vi "HEWH_EnviraCom_Main.vi"(1 "Envira is working":refnum<vi>, 4 "Loop Count":refnum<vi>, 6 "State":refnum<vi>, 8 "error in":errorcluster, 9 "Retry Count":refnum<vi>, 11 "Message Queues out":T1) -> (0 "error out":errorcluster)   [LabVIEW 2023]
uses:
  Tenney/support/Message Queue/All Message Queues.ctl
  Tenney/support/Message Queue/Message Cluster.ctl
  FVIR and LDO/support/Message Queue/Enqueue Message (Single).vi
  FVIR and LDO/support/Message Queue/Message Queue.lvlib
  Tenney/support/Message Queue/Tenney Message Queue.lvlib
panel:
  out "Debug":string[](array[string])
  in  "Debug":bool
  out "Loop Count":i32
  # "Debug"
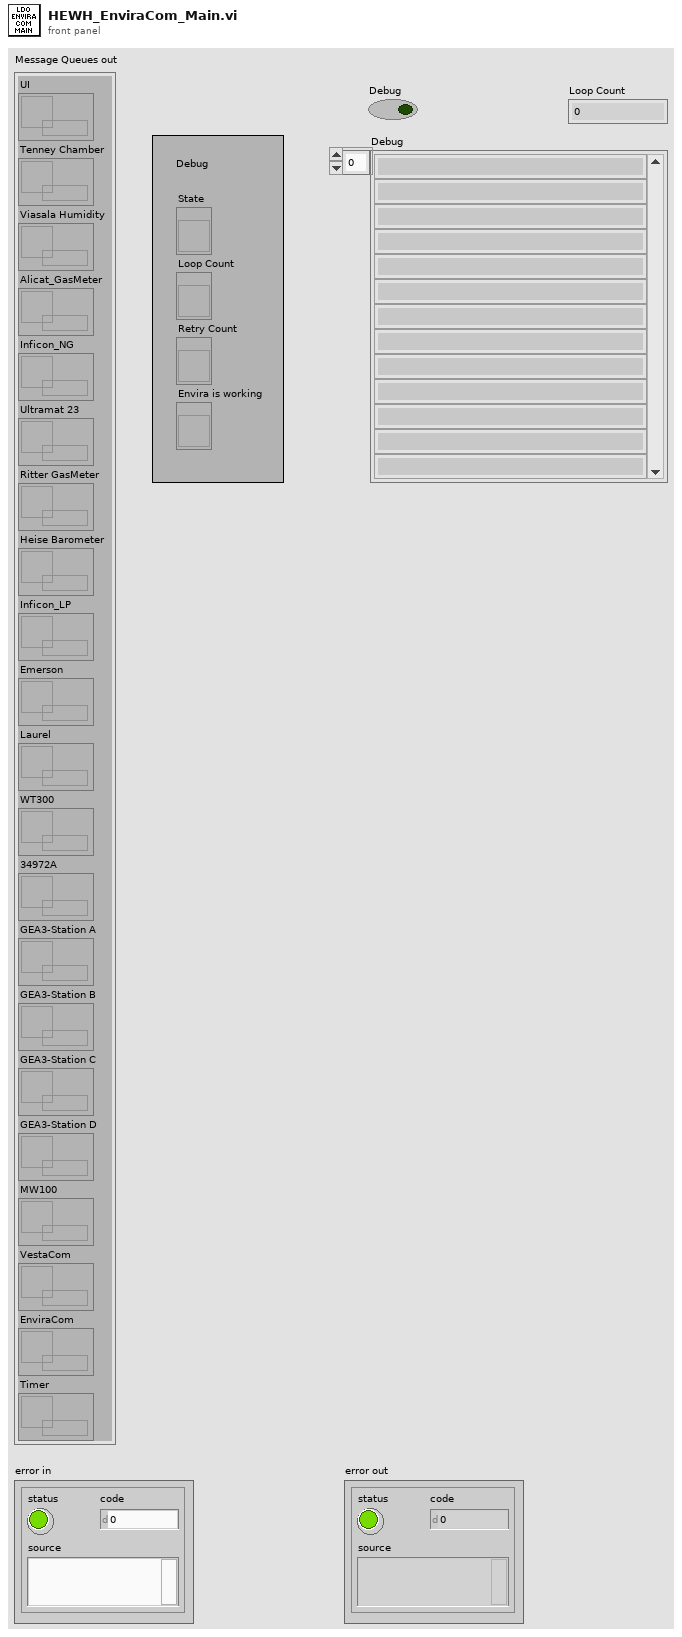
[diagram p1: front panel]
types:
  T1 = typedef "Tenney Message Queue.lvlib/All Message Queues.ctl" = cluster{"UI":refnum<queue>, "Tenney Chamber":refnum<queue>, "Viasala Humidity":refnum<queue>, "Alicat_GasMeter":refnum<queue>, "Inficon_NG":refnum<queue>, "Ultramat 23":refnum<queue>, "Ritter GasMeter":refnum<queue>, "Heise Barometer":refnum<queue>, "Inficon_LP":refnum<queue>, "Emerson":refnum<queue>, "Laurel":refnum<queue>, "WT300":refnum<queue>, "34972A":refnum<queue>, "GEA3-Station A":refnum<queue>, "GEA3-Station B":refnum<queue>, "GEA3-Station C":refnum<queue>, "GEA3-Station D":refnum<queue>, "MW100":refnum<queue>, "VestaCom":refnum<queue>, "EnviraCom":refnum<queue>, "Timer":refnum<queue>}
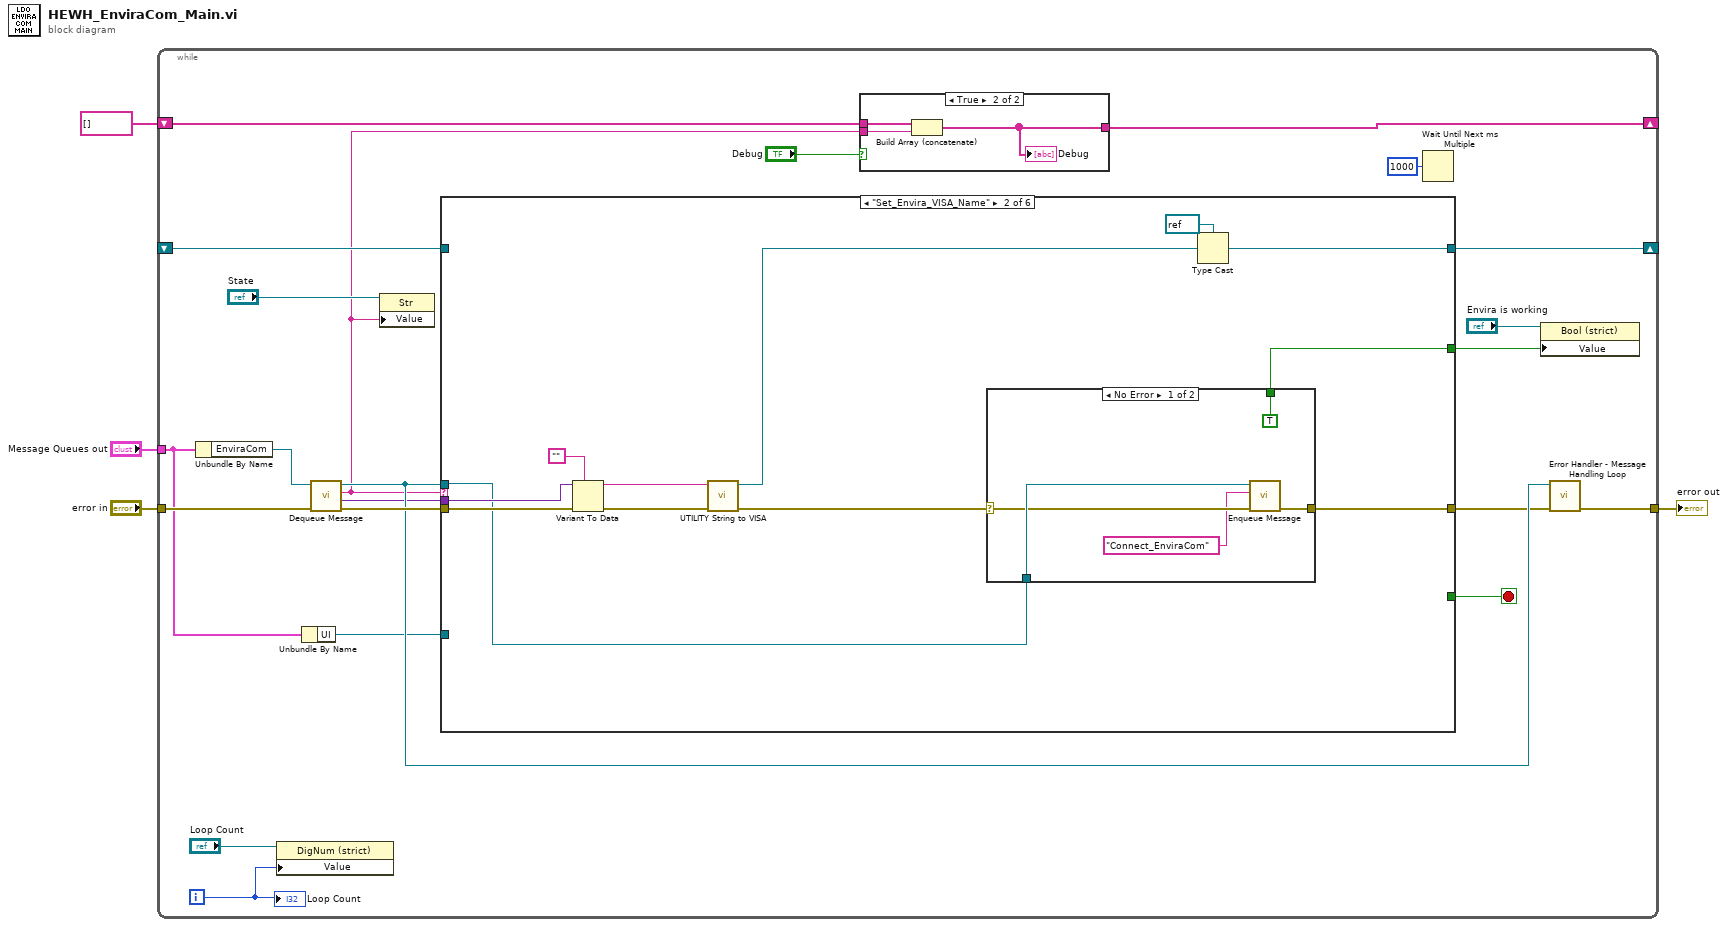
[diagram p0: block diagram]
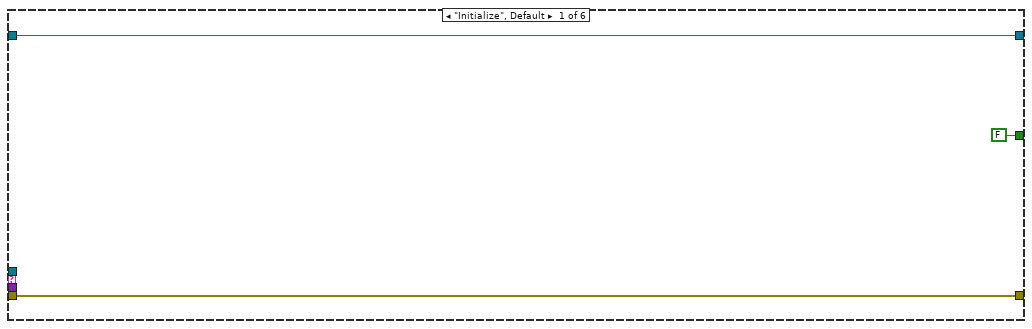
[diagram p3: hidden frame]
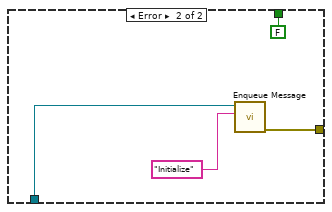
[diagram p4: hidden frame]
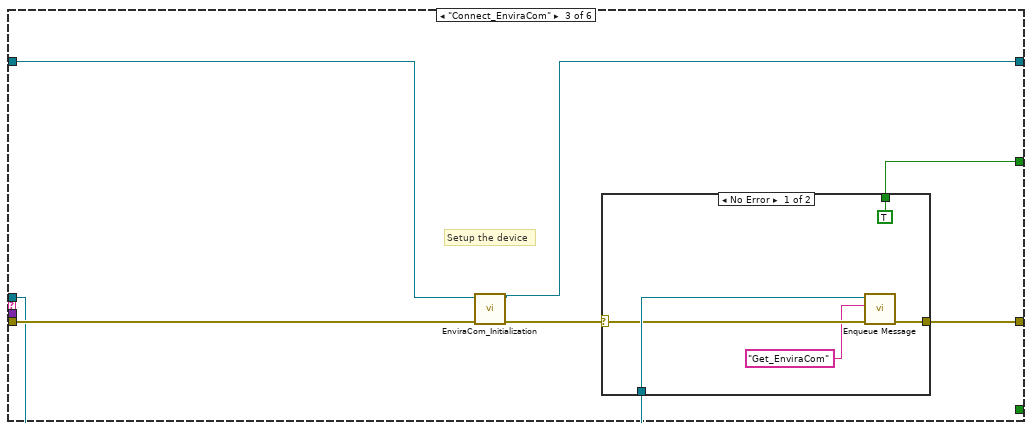
[diagram p5: hidden frame]
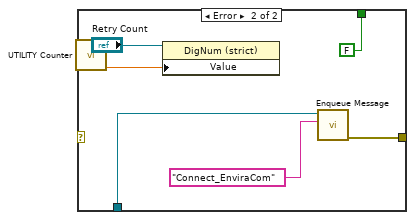
[diagram p6: hidden frame]
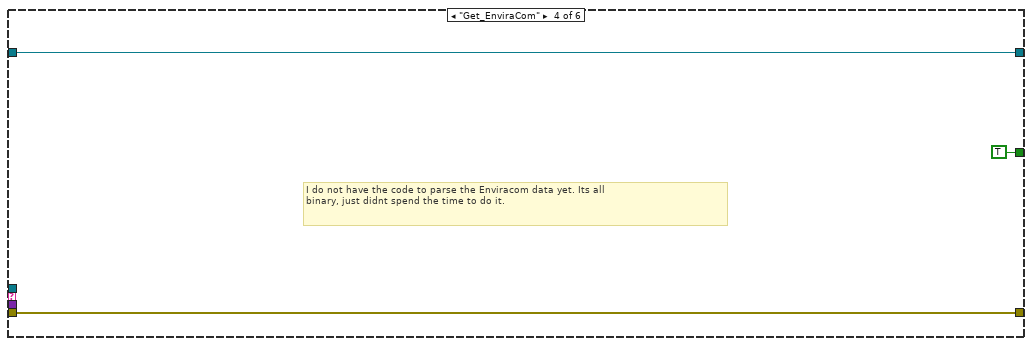
[diagram p7: hidden frame]
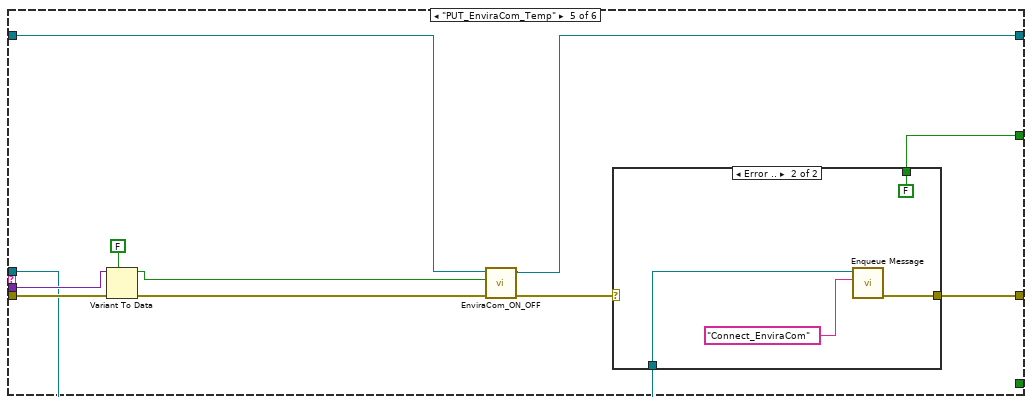
[diagram p8: hidden frame]
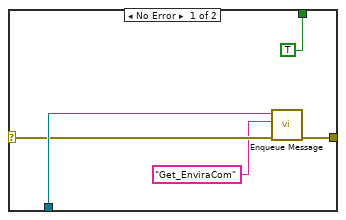
[diagram p9: hidden frame]
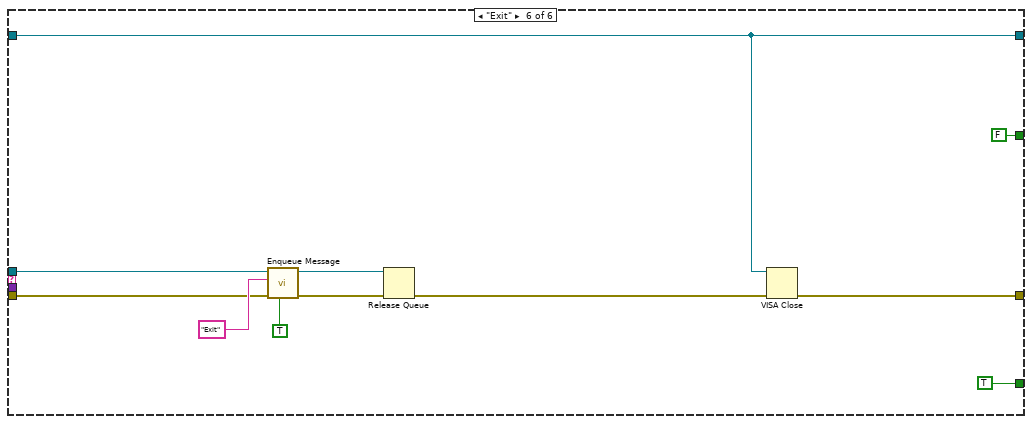
[diagram p10: hidden frame]
diagram:
  n1 = while {
    tunnel: "Message Queues out" -> [w18]
    tunnel: "error in" -> [w25]
    tunnel: [w21] -> w3
    shift-right: [w16] -> _
    shift-left: _ -> [w15]
    shift-right: [w6] -> _
    shift-left: string[] [] -> [w7]
    i -> [w11]
    stop <- w23 stop-if-true
    n2 = Unbundle By Name(w18) -> ("EnviraCom"=w26:refnum<queue>)
    n3 = property class="DigNum (strict)"(reference="Loop Count", "Value"=w11) -> ()  [unwired: 1 in, 2 out]
    n4 = Unbundle By Name(w18) -> ("UI"=w17:refnum<queue>)
    n5 = call "Dequeue Message.vi"("error in (no error)"=w25, "Message Queue"=w26) -> ("error out"=w24:errorcluster, "Message Data"=w14:variant, "Message"=w5:string, "dup Message Queue"=w22:refnum<queue>)  [unwired: 6 in]
    n6 = property class="Str"(reference="State", "Value"=w5) -> ()  [unwired: 1 in, 2 out]
    n7 = case shown="\"Set_Envira_VISA_Name\"" w5 {
      tunnel: w24 -> [w31 w44 w61 w75 w86 w103]
      tunnel: [w31 w39 w58 w75 w78 w99] -> w20
      tunnel: [_ _ _ _ _ TRUE] -> w23
      tunnel: w22 -> [_ w38 w57 _ w77 w97]
      tunnel: w17 -> [_ _ _ _ _ _]
      tunnel: [w33 w34 w59 w74 w82 w98] -> w16
      tunnel: w15 -> [w33 _ w56 w74 w83 w98]
      tunnel: w14 -> [_ w41 _ _ w85 _]
      tunnel: [FALSE ("Vesta Is Working") w35 w55 TRUE ("Vesta Is Working") w76 FALSE ("Vesta Is Working")] -> w9
      frame "Initialize", Default {
      }
      frame "Set_Envira_VISA_Name" {
        n8 = Variant To Data(error in=w44, type="", Variant=w41) -> (data=w42:string, error out=w43:errorcluster)
        n9 = call "UTILITY String to VISA.vi"("error in (no error)"=w43, "VISA Name"=w42) -> ("error out"=w40:errorcluster, "VISA resource name out"=w37:refnum<visa-resource-name>)  [unwired: 8 in]
        n10 = case shown="No Error" w40 {
          selector: w40 -> [w48 _]
          tunnel: [w50 w54] -> w39
          tunnel: w38 -> [w49 w53]
          tunnel: [TRUE ("Vesta Is Working") FALSE ("Vesta Is Working")] -> w35
          frame No Error {
            n11 = call-poly "Enqueue Message.vi"("error in (no error)"=w48, "Message"="Connect_EnviraCom", "Message Queue"=w49) -> ("error out"=w50:errorcluster)  [unwired: 7 in, 1 out]
          }
          frame Error {
            n12 = call-poly "Enqueue Message.vi"("Message"="Initialize", "Message Queue"=w53) -> ("error out"=w54:errorcluster)  [unwired: 8 in, 1 out]
          }
        }
        n13 = Type Cast(type=refnum<visa-resource-name> refnum ("VISA resource name"), x=w37) -> (*(type *) &x=w34:refnum<visa-resource-name>)
      }
      frame "Connect_EnviraCom" {
        # "Setup the device"
        n14 = call "EnviraCom_Initialization.vi"("error in (no error)"=w61, "VISA Refnum in"=w56) -> ("error out"=w60:errorcluster, "VISA Refnum out"=w59:refnum<visa-resource-name>)  [unwired: 8 in]
        n15 = case shown="No Error" w60 {
          selector: w60 -> [w64 _]
          tunnel: [w66 w70] -> w58
          tunnel: w57 -> [w65 w69]
          tunnel: [TRUE ("Vesta Is Working") FALSE ("Vesta Is Working")] -> w55
          frame No Error {
            n16 = call-poly "Enqueue Message.vi"("error in (no error)"=w64, "Message"="Get_EnviraCom", "Message Queue"=w65) -> ("error out"=w66:errorcluster)  [unwired: 7 in, 1 out]
          }
          frame Error {
            n17 = call "UTILITY Counter.vi"() -> ("Count"=w72:dbl)  [unwired: 11 in]
            n18 = property class="DigNum (strict)"(reference="Retry Count", "Value"=w72) -> ()  [unwired: 1 in, 2 out]
            n19 = call-poly "Enqueue Message.vi"("Message"="Connect_EnviraCom", "Message Queue"=w69) -> ("error out"=w70:errorcluster)  [unwired: 8 in, 1 out]
          }
        }
      }
      frame "Get_EnviraCom" {
        # "I do not have the code to parse the Enviracom data yet. Its all\nbinary, just didnt spend the time to do it."
      }
      frame "PUT_EnviraCom_Temp" {
        n20 = Variant To Data(error in=w86, type=FALSE, Variant=w85) -> (data=w80:bool, error out=w84:errorcluster)
        n21 = call "EnviraCom_ON_OFF.vi"("error in (no error)"=w84, "ON (True), OFF (False)"=w80, "VISA Refnum in"=w83) -> ("error out"=w79:errorcluster, "VISA Refnum out"=w82:refnum<visa-resource-name>)  [unwired: 7 in]
        n22 = case shown="Error .." w79 {
          selector: w79 -> [w89 _]
          tunnel: [w91 w95] -> w78
          tunnel: w77 -> [w90 w94]
          tunnel: [TRUE ("Vesta Is Working") FALSE ("Vesta Is Working")] -> w76
          frame No Error {
            n23 = call-poly "Enqueue Message.vi"("error in (no error)"=w89, "Message"="Get_EnviraCom", "Message Queue"=w90) -> ("error out"=w91:errorcluster)  [unwired: 7 in, 1 out]
          }
          frame Error {
            n24 = call-poly "Enqueue Message.vi"("Message"="Connect_EnviraCom", "Message Queue"=w94) -> ("error out"=w95:errorcluster)  [unwired: 8 in, 1 out]
          }
        }
      }
      frame "Exit" {
        n25 = call-poly "Enqueue Message.vi"("Priority Message? (F)"=TRUE, "error in (no error)"=w103, "Message"="Exit", "Message Queue"=w97) -> ("error out"=w102:errorcluster, "dup Message Queue"=w96:refnum<queue>)  [unwired: 6 in]
        n26 = Release Queue(queue=w96, error in (no error)=w102) -> (error out=w100:errorcluster)  [unwired: 1 in, 2 out]
        n27 = VISA Close(VISA resource name=w98, error in (no error)=w100) -> (error out=w99:errorcluster)
      }
    }
    n28 = case shown="True" "Debug" {
      tunnel: w5 -> [_ w30]
      tunnel: w7 -> [w27 w29]
      tunnel: [w27 w28] -> w6
      frame False {
      }
      frame True {
        n29 = Build Array (concatenate)(w29, w30) -> (w28:string[])
        "Debug" <- w28
      }
    }
    n30 = Wait Until Next ms Multiple(millisecond multiple=u32 1000) -> ()  [unwired: 1 out]
    n31 = property class="Bool (strict)"(reference="Envira is working", "Value"=w9) -> ()  [unwired: 1 in, 2 out]
    n32 = call "Error Handler - Message Handling Loop.vi"("error in (no error)"=w20, "Message Queue"=w22) -> ("dup error in"=w21:errorcluster)  [unwired: 8 in, 1 out]
    "Loop Count" <- w11
  }
  "error out" <- w3
